vi "Sort Control Refs.vi"(8 "error in (no error)":errorcluster, 10 "Terminal Bounds[]":T1[](array[typedef]), 11 "Unsorted Refnums":refnum<vi>[](array[refnum])) -> (0 "error out":errorcluster, 1 "Sorted Control Indices":i32[](array[numeric]), 2 "Sorted Controls":refnum<vi>[](array[refnum]), 4 "Sorted Indicators":refnum<vi>[](array[refnum]), 6 "Sorted Indicator Indices":i32[](array[numeric]))   [LabVIEW 2020, in "Message Maker.lvlib"]
uses:
  Message Maker.lvlib
  <vilib>/Utility/miscctls.llb/LVRectTypeDef.ctl
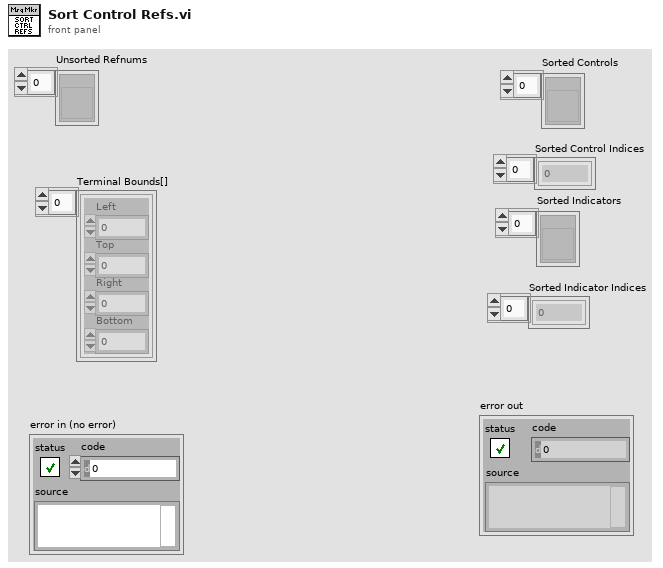
[diagram p1: front panel]
types:
  T1 = typedef "LVRectTypeDef.ctl" = cluster{"Left":i16, "Top":i16, "Right":i16, "Bottom":i16}
  T2 = cluster{"Index":i32, "Control Ref":refnum<vi>, "Term Bounds":T1}[]
  T3 = cluster{i32, "Ctl Refnum":refnum<vi>, "Rectangle":T1}
  T4 = cluster{"Index":i32, "Ctl Refnum":refnum<vi>, "Rectangle":T1}[]
  T5 = cluster{"Top":i16, "Left":i16, cluster{"Index":i32, "Control Ref":refnum<vi>, "Term Bounds":T1}}
  T6 = cluster{"Top":i16, "Left":i16, cluster{"Index":i32, "Control Ref":refnum<vi>, "Term Bounds":T1}}[]
  T7 = cluster{"Index":i32, "Control Ref":refnum<vi>, "Term Bounds":T1}
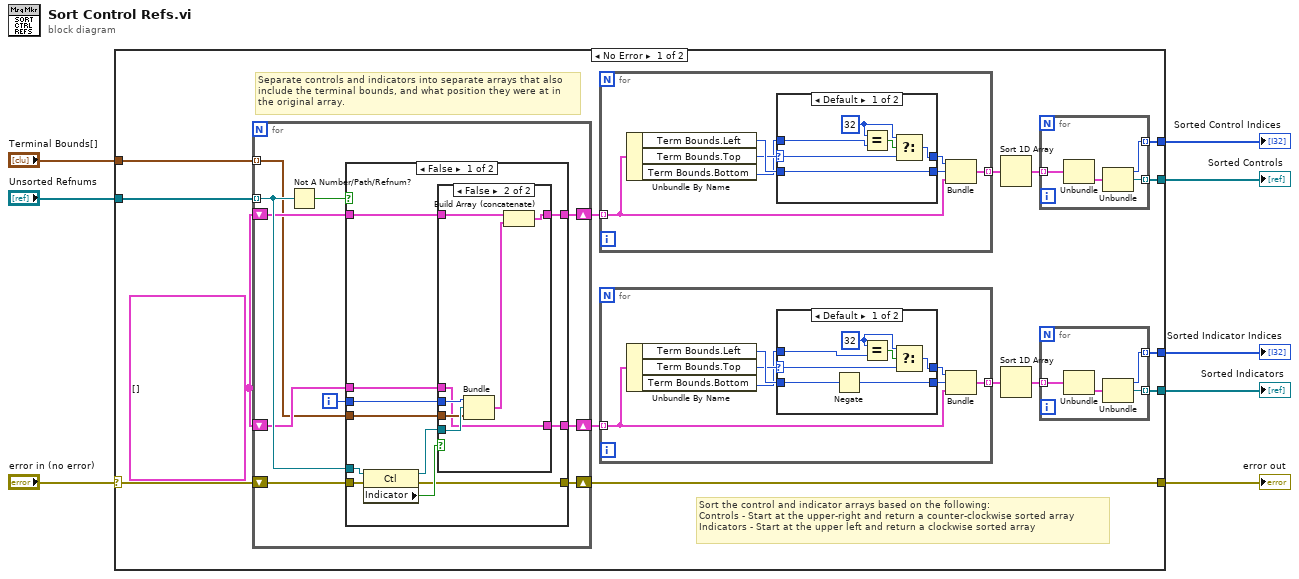
[diagram p0: block diagram]
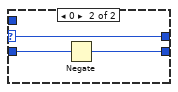
[diagram p3: hidden frame]
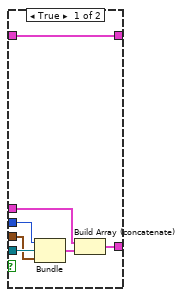
[diagram p4: hidden frame]
diagram:
  n1 = case shown="No Error" "error in (no error)" {
    selector: "error in (no error)" -> [w14 w102]
    tunnel: "Unsorted Refnums" -> [w16 _]
    tunnel: "Terminal Bounds[]" -> [w15 _]
    tunnel: [w13 w102] -> w5
    tunnel: [w12 _] -> w4
    tunnel: [w11 _] -> w3
    tunnel: [w10 _] -> w2
    tunnel: [w9 _] -> w1
    frame No Error {
      w23 = T2 []
      # "Sort the control and indicator arrays based on the following:\nControls - Start at the upper-right and return a counter-clockwise sorted array\nIndicators - Start at the upper left and return a clockwise sorted array"
      # "Separate controls and indicators into separate arrays that also include the terminal bounds, and what position they were at in the original array."
      n2 = for {
        shift-right: [w70] -> w13
        shift-left: w14 -> [w73]
        tunnel: w16 -> [w71] mode=indexing
        shift-right: [w67] -> w22
        shift-left: w23 -> [w69]
        shift-right: [w66] -> w19
        shift-left: w23 -> [w68]
        tunnel: w15 -> [w64] mode=indexing
        i -> [w65]
        n3 = Not A Number/Path/Refnum?(number/path/refnum=w71) -> (NaN/Path/Refnum?=w72:bool)
        n4 = case shown="False" w72 {
          tunnel: w73 -> [w84 w101]
          tunnel: w71 -> [w83 _]
          tunnel: [w79 w101] -> w70
          tunnel: w69 -> [w81 w100]
          tunnel: w68 -> [w80 w99]
          tunnel: [w78 w100] -> w67
          tunnel: [w77 w99] -> w66
          tunnel: w65 -> [w76 _]
          tunnel: w64 -> [w74 _]
          frame False {
            n5 = property class="Ctl"(reference=w83, error in=w84) -> (reference out=w75:refnum<vi>, error out=w79:errorcluster, "Indicator"=w82:bool)
            n6 = case shown="False" w82 {
              tunnel: w81 -> [w91 w93]
              tunnel: w80 -> [w90 w92]
              tunnel: [w91 w94] -> w78
              tunnel: [w89 w92] -> w77
              tunnel: w76 -> [w88 w98]
              tunnel: w75 -> [w87 w97]
              tunnel: w74 -> [w86 w96]
              frame True {
                n7 = Bundle(w88, "Ctl Refnum"=w87, "Rectangle"=w86) -> (w85:T3)  [unwired: 1 in]
                n8 = Build Array (concatenate)(w90, w85) -> (w89:T4)
              }
              frame False {
                n9 = Bundle(w98, "Ctl Refnum"=w97, "Rectangle"=w96) -> (w95:T3)  [unwired: 1 in]
                n10 = Build Array (concatenate)(w93, w95) -> (w94:T4)
              }
            }
          }
          frame True {
          }
        }
      }
      n11 = for {
        tunnel: w22 -> [w51] mode=indexing
        tunnel: [w50] -> w21 mode=indexing
        n12 = Unbundle By Name(w51) -> ("Term Bounds.Left"=w54:i16, "Term Bounds.Top"=w52:i16, "Term Bounds.Bottom"=w48:i16)
        n13 = case shown="Default" w52 {
          selector: w52 -> [w56 w61]
          tunnel: w54 -> [w60 w63]
          tunnel: [w60 w62] -> w53
          tunnel: [w55 w61] -> w49
          tunnel: w48 -> [w59 _]
          frame Default {
            w57 = i16 32 ("x")
            n14 = Equal?(x=w57, y=w59) -> (x = y?=w58:bool)
            n15 = Select(t=w57, s=w58, f=w56) -> (s? t:f=w55:i16)
          }
          frame 0 {
            n16 = Negate(x=w63) -> (-x=w62:i16)
          }
        }
        n17 = Bundle("Top"=w49, "Left"=w53, w51) -> (w50:T5)  [unwired: 1 in]
      }
      n18 = for {
        tunnel: w19 -> [w31] mode=indexing
        tunnel: [w30] -> w17 mode=indexing
        n19 = Unbundle By Name(w31) -> ("Term Bounds.Left"=w34:i16, "Term Bounds.Top"=w32:i16, "Term Bounds.Bottom"=w28:i16)
        n20 = case shown="Default" w32 {
          selector: w32 -> [w37 w42]
          tunnel: w34 -> [w41 w43]
          tunnel: [w35 w43] -> w33
          tunnel: [w36 w42] -> w29
          tunnel: w28 -> [w40 _]
          frame Default {
            w38 = i16 32 ("x")
            n21 = Negate(x=w41) -> (-x=w35:i16)
            n22 = Equal?(x=w38, y=w40) -> (x = y?=w39:bool)
            n23 = Select(t=w38, s=w39, f=w37) -> (s? t:f=w36:i16)
          }
          frame 0 {
          }
        }
        n24 = Bundle("Top"=w29, "Left"=w33, w31) -> (w30:T5)  [unwired: 1 in]
      }
      n25 = Sort 1D Array(array=w21) -> (sorted array=w20:T6)
      n26 = Sort 1D Array(array=w17) -> (sorted array=w18:T6)
      n27 = for {
        tunnel: w20 -> [w47] mode=indexing
        tunnel: [w45] -> w10 mode=indexing
        tunnel: [w44] -> w12 mode=indexing
        n28 = Unbundle(w47) -> (w46:T7)  [unwired: 2 out]
        n29 = Unbundle(w46) -> ("Index"=w45:i32, "Control Ref"=w44:refnum<vi>)  [unwired: 1 out]
      }
      n30 = for {
        tunnel: w18 -> [w27] mode=indexing
        tunnel: [w25] -> w9 mode=indexing
        tunnel: [w24] -> w11 mode=indexing
        n31 = Unbundle(w27) -> (w26:T7)  [unwired: 2 out]
        n32 = Unbundle(w26) -> ("Index"=w25:i32, "Control Ref"=w24:refnum<vi>)  [unwired: 1 out]
      }
    }
    frame Error {
    }
  }
  "Sorted Controls" <- w4
  "Sorted Indicators" <- w3
  "error out" <- w5
  "Sorted Control Indices" <- w2
  "Sorted Indicator Indices" <- w1
